vi "SetShutter.vi"(8 "error in (no error)":errorcluster, 10 "State":bool, 11 "Topas":refnum<k24>) -> (0 "error out":errorcluster, 3 "Topas Out":refnum<k24>)   [LabVIEW 2017]
uses:
  D:/upwork/Laser Measurement Tool/Topas4PublicAPI/NET_SDK/Topas4Lib.dll
  Topas4PublicAPI/NET_SDK/Topas4Lib.dll
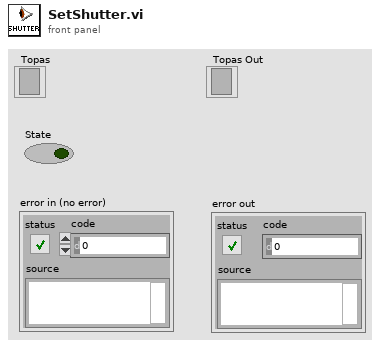
[diagram p1: front panel]
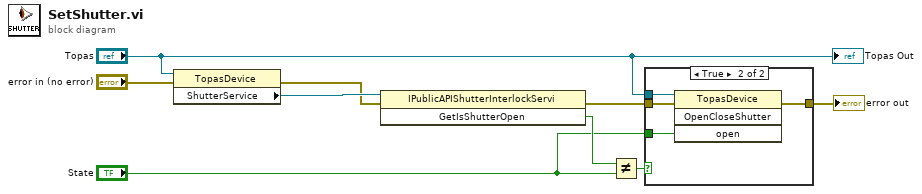
[diagram p0: block diagram]
diagram:
  n1 = property class="TopasDevice"(reference="Topas", error in="error in (no error)") -> (error out=w6:errorcluster, "ShutterService"=w8:refnum<k24>)  [unwired: 1 out]
  n2 = invoke class="IPublicAPIShutterInterlockServi" method="GetIsShutterOpen"(reference=w8, error in=w6) -> (error out=w5:errorcluster, "GetIsShutterOpen"=w3:bool)  [unwired: 1 in, 1 out]
  n3 = Not Equal?(x=w3, y="State") -> (x != y?=w2:bool)
  n4 = case shown="True" w2 {
    tunnel: "Topas" -> [_ w14]
    tunnel: w5 -> [w10 w13]
    tunnel: [w10 w12] -> w4
    tunnel: "State" -> [_ w11]
    frame False {
    }
    frame True {
      n5 = invoke class="TopasDevice" method="OpenCloseShutter"(reference=w14, error in=w13, "open"=w11) -> (error out=w12:errorcluster)  [unwired: 1 in, 3 out]
    }
  }
  "error out" <- w4
  "Topas Out" <- "Topas"
